vi "sub_checksum.vi"(9 "NMEA String (~\\n이전)":string) -> (1 "equal?":bool, 2 "raw checksum":string, 3 "cal checksum":string)   [LabVIEW 2020]
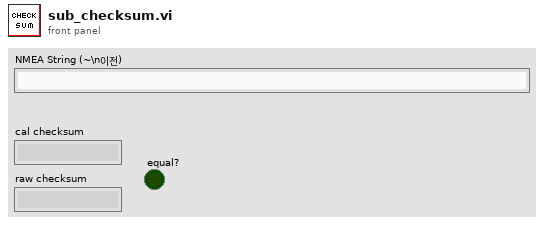
[diagram p1: front panel]
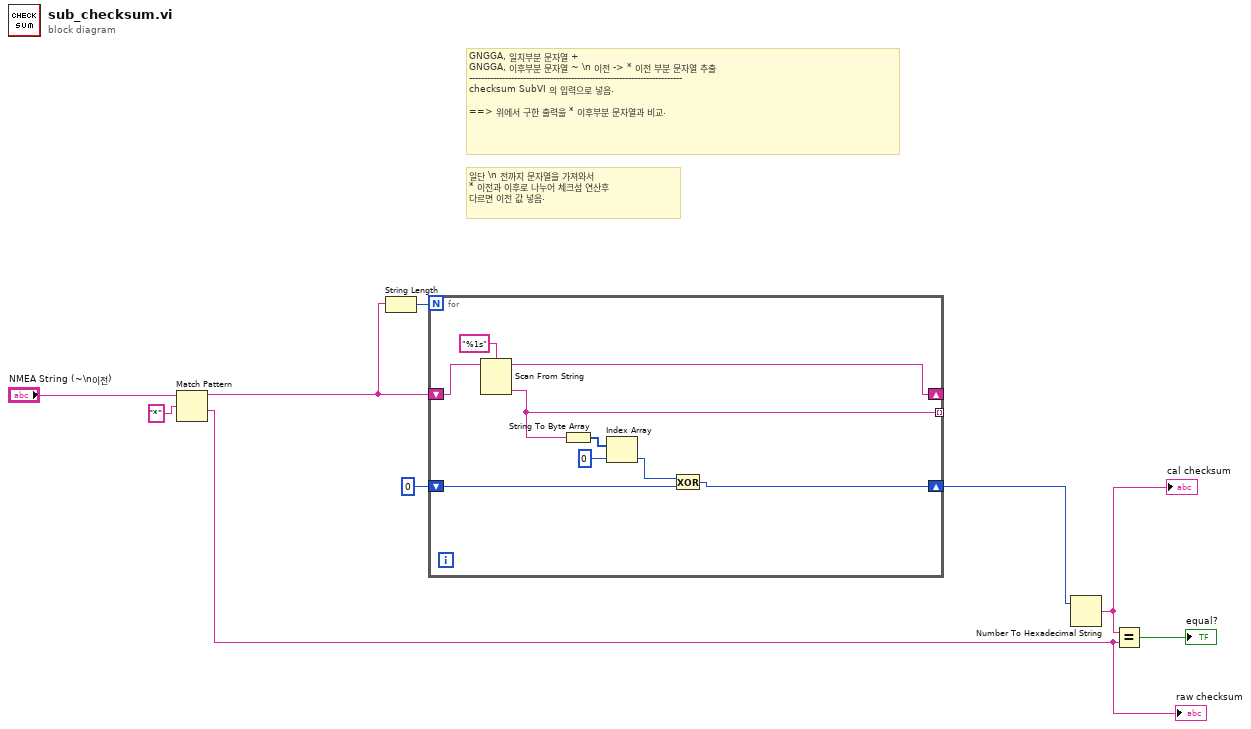
[diagram p0: block diagram]
diagram:
  # "GNGGA, 일치부분 문자열 + \nGNGGA, 이후부분 문자열 ~ \\n 이전 -> * 이전 부분 문자열 추출\n-----------------------------------------------------------------------\nchecksum SubVI 의 입력으로 넣음.\n\n==> 위에서 구한 출력을 * 이후부분 문자열과 비교."
  # "일단 \\n 전까지 문자열을 가져와서\n* 이전과 이후로 나누어 체크섬 연산후\n다르면 이전 값 넣음."
  n1 = Match Pattern(string="NMEA String (~\\n이전)", regular expression="*" ("정규식")) -> (before substring=w1:string, after substring=w7:string)  [unwired: 1 in, 2 out]
  "raw checksum" <- w7
  n2 = String Length(string=w1) -> (length=w2:i32)
  n3 = for {
    N: w2 -> [_]
    shift-right: [w16] -> _
    shift-left: w1 -> [w18]
    tunnel: [w15] -> _ mode=indexing
    shift-right: [w11] -> w6
    shift-left: u8 0 -> [w12]
    n4 = Scan From String(format string="%1s" ("포맷 문자열"), input string=w18) -> (remaining string=w16:string, output 1=w15:string)  [unwired: 3 in, 2 out]
    n5 = String To Byte Array(string=w15) -> (unsigned byte array=w14:u8[])
    n6 = Index Array(array=w14, index=0 ("인덱스")) -> (element=w10:u8)
    n7 = Exclusive Or(1:w12, 2:w10) -> (0:w11:u8)
  }
  n8 = Number To Hexadecimal String(2:w6) -> (0:w3:string)  [unwired: 1 in]
  "cal checksum" <- w3
  n9 = Equal?(x=w3, y=w7) -> (x = y?=→"equal?":bool)
